vi "ActionVIOnDelete.vi"(6 "All deleted Refs":T1[](array[typedef]) format="%.0x", 8 "error in (no error)":errorcluster, 11 "Item Ref in":T1 format="%.0x") -> (0 "error out":errorcluster, 3 "Item Ref out":T1 format="%.0x")   [LabVIEW 2015, in "Protection and Counter Addon System Explorer.lvlib"]
uses:
  Protection and Counter Addon System Explorer.lvlib
  <vilib>/NI Veristand/Custom Device API/Custom Device Item Ref.ctl
  <vilib>/NI Veristand/Custom Device Tools/Custom Device Utility Library/NI VeriStand - Search for Item by GUID.vi
  <vilib>/NI Veristand/Custom Device Tools/Custom Device Utility Library/NI VeriStand - Search for Item by Name.vi
  <vilib>/NI VeriStand/Custom Device Tools/Custom Device Utility Library/Custom Device Utility Library.lvlib
  <vilib>/NI VeriStand/Custom Device API/Custom Device API.lvlib
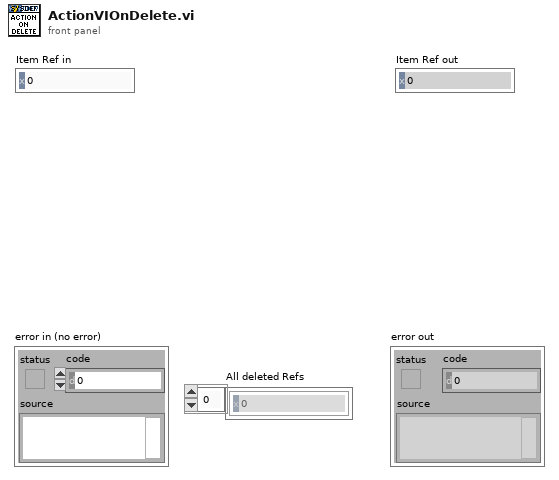
[diagram p1: front panel]
types:
  T1 = typedef "Custom Device API.lvlib/Custom Device Item Ref.ctl" = u64
  T2 = typedef "Protection and Counter Addon Shared.lvlib/XNET Settings.ctl" = cluster{"Database":refnum<k21>, "Cluster":refnum<k21>, "Port":string, "Baud rate [Bd]":u64, "Termination":u32, "CAN I/O Mode":u32, "FD Baud rate [Bd]":u64, "Priority":i32, "Use Legacy":bool}
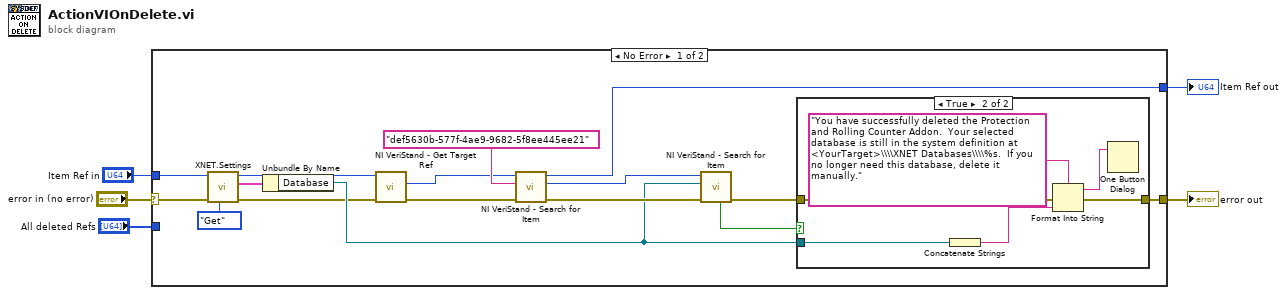
[diagram p0: block diagram]
diagram:
  n1 = case shown="No Error" "error in (no error)" {
    selector: "error in (no error)" -> [w21 w30]
    tunnel: [w19 w30] -> w4
    tunnel: "Item Ref in" -> [w20 w29]
    tunnel: [w18 w29] -> w2
    tunnel: "All deleted Refs" -> [_ _]
    frame No Error {
      n2 = call "XNET.Settings.vi"("Action"=enum8{"Get", "Set"}."Get", "error in (no error)"=w21, "Parent Ref in"=w20) -> ("error out"=w7:errorcluster, "XNET Settings"=w8:T2, "Item Ref out"=w12:T1)  [unwired: 6 in]
      n3 = Unbundle By Name(w8) -> ("Database"=w9:refnum<k21>)
      n4 = call <vilib>:"NI VeriStand - Get Target Ref.vi"("error in"=w7, "Item Ref in"=w12) -> ("error out"=w10:errorcluster, "Target Ref"=w11:T1)  [unwired: 6 in, 2 out]
      n5 = call-poly <vilib>:"NI VeriStand - Search for Item.vi"("error in"=w10, "Item GUID"="def5630b-577f-4ae9-9682-5f8ee445ee21" ("string"), "Section Ref in"=w11) -> ("error out"=w15:errorcluster, "Item Ref"=w16:T1, "Section Ref out"=w18:T1)  [unwired: 5 in, 1 out]
      n6 = call-poly <vilib>:"NI VeriStand - Search for Item.vi"("error in"=w15, "Item Name"=w9, "Section Ref in"=w16) -> ("error out"=w14:errorcluster, "Found"=w13:bool)  [unwired: 5 in, 2 out]
      n7 = case shown="True" w13 {
        tunnel: w14 -> [w22 w28]
        tunnel: [w22 w27] -> w19
        tunnel: w9 -> [_ w24]
        frame False {
        }
        frame True {
          n8 = Concatenate Strings(w24) -> (w23:string)
          n9 = Format Into String(format string="You have successfully deleted the Protection and Rolling Counter Addon.  Your selected database is still in the system definition at <YourTarget>\\\\XNET Databases\\\\%s.  If you no longer need this database, delete it manually." ("message"), error in=w28, w23) -> (resulting string=w25:string, error out=w27:errorcluster)  [unwired: 1 in]
          n10 = One Button Dialog(message=w25) -> ()  [unwired: 1 in, 1 out]
        }
      }
    }
    frame Error {
    }
  }
  "error out" <- w4
  "Item Ref out" <- w2
